vi "basics.vi"() -> ()   [LabVIEW 2020]
panel:
  out "Meter":dbl(knob) scale=0.0..10.0
  out "Slide":u8(slide) scale=0.0..100.0
  out "Gauge":dbl(knob) scale=0.0..10.0
  out "Thermometer":dbl(slide) scale=0.0..10.0
  out "Tank":dbl(slide) scale=0.0..10.0
  in  "Numeric":dbl
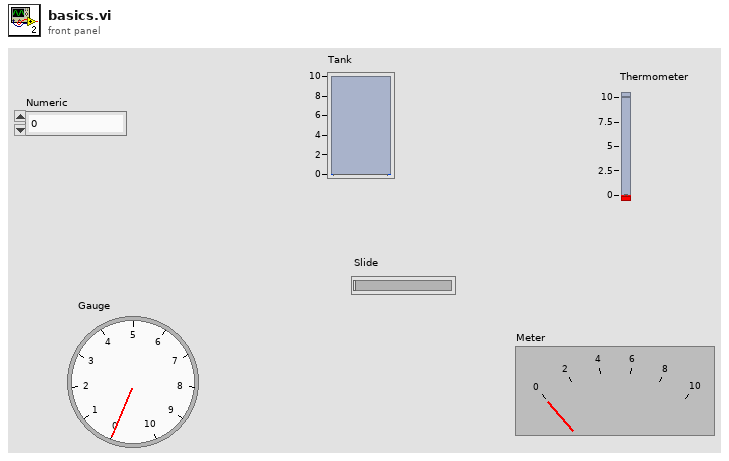
[diagram p1: front panel]
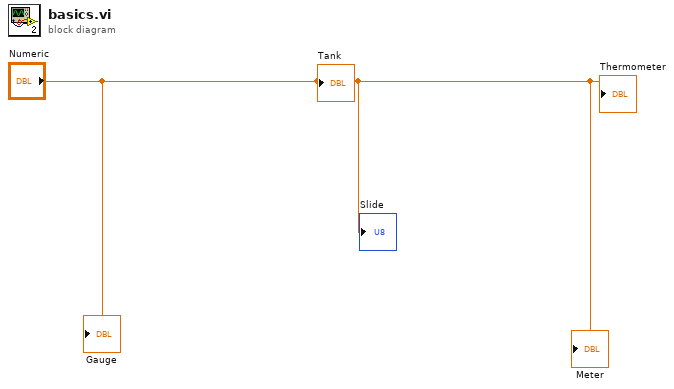
[diagram p0: block diagram]
diagram:
  "Tank" <- "Numeric"
  "Thermometer" <- "Numeric"
  "Gauge" <- "Numeric"
  "Slide" <- "Numeric"
  "Meter" <- "Numeric"
